vi "Split auto name from auto program.vi"(11 "Programs with names":string[](array[string])) -> (2 "Programs":string[](array[string]), 3 "Program Name":string[](array[string]))   [LabVIEW 2013]
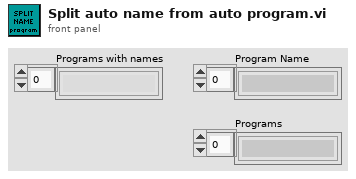
[diagram p1: front panel]
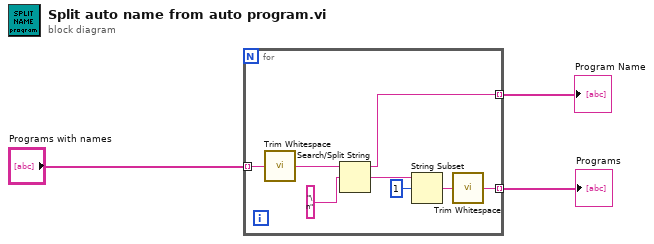
[diagram p0: block diagram]
diagram:
  n1 = for {
    tunnel: "Programs with names" -> [w6] mode=indexing
    tunnel: [w11] -> w1 mode=indexing
    tunnel: [w4] -> w2 mode=indexing
    n2 = call <vilib>:"Trim Whitespace.vi"("string"=w6) -> ("trimmed string"=w5:string)  [unwired: 1 in]
    n3 = Search/Split String(string=w5, search string/char (-)="\n") -> (substring before match=w11:string, match + rest of string=w10:string)  [unwired: 1 in, 1 out]
    n4 = String Subset(string=w10, offset (0)=1) -> (substring=w9:string)  [unwired: 1 in]
    n5 = call <vilib>:"Trim Whitespace.vi"("string"=w9) -> ("trimmed string"=w4:string)  [unwired: 1 in]
  }
  "Programs" <- w2
  "Program Name" <- w1
